vi "centered_gauss_3.vi"() -> ()   [LabVIEW 2016]
panel:
  out "exp(x)":dbl
  in  "time":dbl
  out "output":dbl
  in  "Frequency(MHz)":dbl
  in  "Pulse Spacing":dbl
  in  "Amplitude":dbl
  in  "Envelope DecayTime(micro s)":dbl
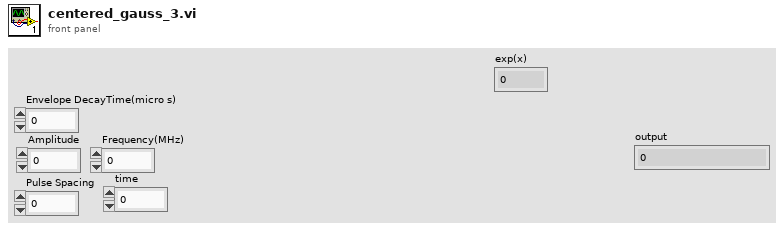
[diagram p1: front panel]
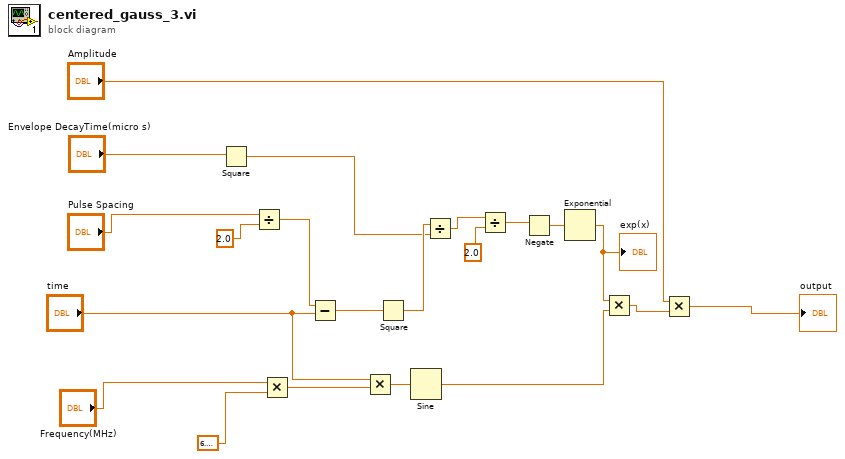
[diagram p0: block diagram]
diagram:
  n1 = Square(x="Envelope DecayTime(micro s)") -> (x^2=w12:dbl)
  n2 = Divide(x="Pulse Spacing", y=2.0) -> (x/y=w15:dbl)
  n3 = Multiply(x="Frequency(MHz)", y=6.283185307179586) -> (x*y=w14:dbl)
  n4 = Subtract(x=w15, y="time") -> (x-y=w16:dbl)
  n5 = Multiply(x="time", y=w14) -> (x*y=w6:dbl)
  n6 = Square(x=w16) -> (x^2=w13:dbl)
  n7 = Sine(x=w6) -> (sin(x)=w9:dbl)
  n8 = Divide(x=w13, y=w12) -> (x/y=w4:dbl)
  n9 = Divide(x=w4, y=2.0) -> (x/y=w5:dbl)
  n10 = Negate(x=w5) -> (-x=w11:dbl)
  n11 = Exponential(1:w11) -> (0:w10:dbl)
  "exp(x)" <- w10
  n12 = Multiply(x=w10, y=w9) -> (x*y=w1:dbl)
  n13 = Multiply(x="Amplitude", y=w1) -> (x*y=→"output":dbl)
